vi "GetValueString.vi"(7 "LabVIEW Web Service Request":refnum<class "Web Request.lvclass">, 11 "ControlName":string="Start") -> (1 "Error":i32, 2 "ErrorString":string, 3 "dataOut":string)   [LabVIEW 2024]
uses:
  <vilib>/wsapi/Web Request.lvclass
  g_VIServerPort.vi
panel:
  out "value":string
  out "errorOut":errorcluster
  # "Use the Web Service Request input terminal to call the VIs on the Web Services palette. Do not remove it from the connector pane unless you don't need access to the palette."
  # "Each additional control wired to the connector pane will be available as an input in the URL. To include an indicator in terminal-mode output (the default setting), it must also be wired to the connector pane."
  # "http://127.0.0.1:8002/WebService/GetValueString?ControlName=MPBID_s"
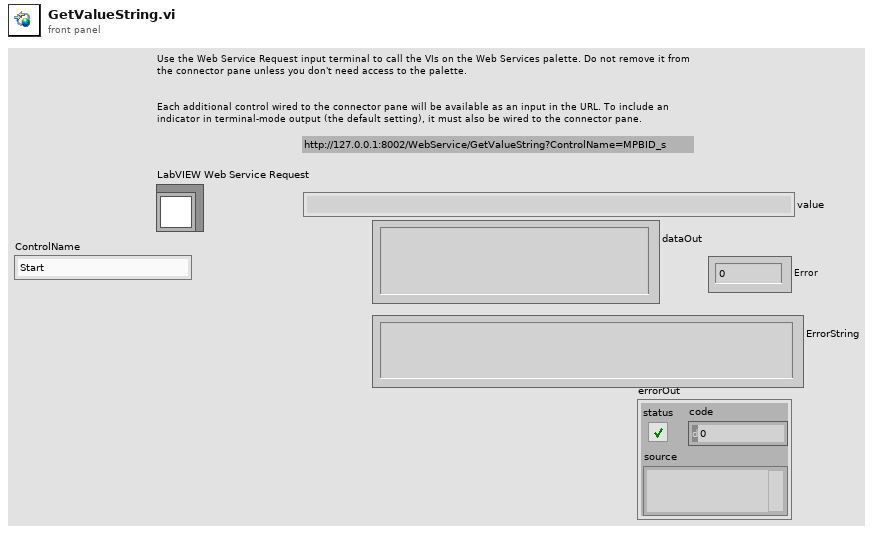
[diagram p1: front panel]
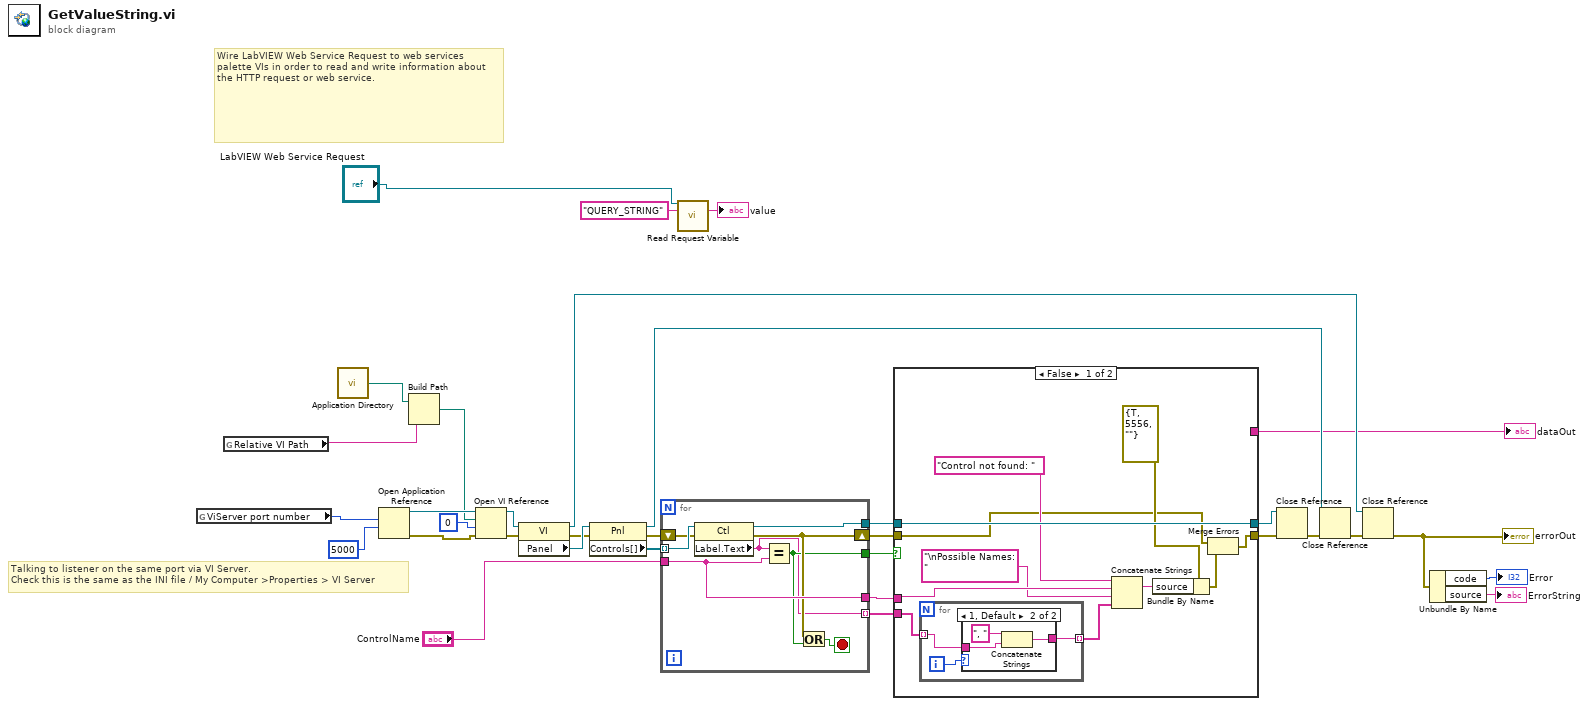
[diagram p0: block diagram]
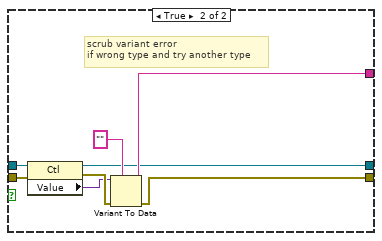
[diagram p3: hidden frame]
diagram:
  # "Talking to listener on the same port via VI Server.\nCheck this is the same as the INI file / My Computer >Properties > VI Server"
  # "Wire LabVIEW Web Service Request to web services palette VIs in order to read and write information about the HTTP request or web service."
  n1 = global read "g_VIServerPort.vi" "ViServer port number"() -> (w2:u16)
  n2 = global read "g_VIServerPort.vi" "Relative VI Path"() -> (w1:string)
  n3 = call <vilib>:"Application Directory.vi"() -> ("Application Directory"=w8:path)
  n4 = Open Application Reference(9:5000 ("timeout ms (60000)"), 10:w2) -> (0:w14:errorcluster, 3:w15:refnum<vi>)  [unwired: 2 in]
  n5 = Build Path(base path=w8, name or relative path=w1) -> (appended path=w7:path)
  n6 = Open VI Reference(application reference (local)=w15, vi path=w7, options=0, error in (no error)=w14) -> (vi reference=w17:refnum<vi>, error out=w29:errorcluster)  [unwired: 2 in]
  n7 = property class="VI"(reference=w17, error in=w29) -> (reference out=w24:refnum<vi>, error out=w28:errorcluster, "Panel"=w32:refnum<vi>)
  n8 = property class="Pnl"(reference=w32, error in=w28) -> (reference out=w18:refnum<vi>, error out=w27:errorcluster, "Controls[]"=w31:refnum<vi>[])
  n9 = for {
    tunnel: w31 -> [w41] mode=indexing
    tunnel: "ControlName" -> [w38]
    tunnel: [w35] -> w26
    tunnel: [w39] -> w19
    tunnel: [w38] -> w16
    shift-right: [w36] -> w20
    shift-left: w27 -> [w40]
    tunnel: [w34] -> w10 mode=indexing
    stop <- w37 stop-if-true
    n10 = property class="Ctl"(reference=w41, error in=w40) -> (reference out=w39:refnum<vi>, error out=w36:errorcluster, "Label.Text"=w34:string)
    n11 = Equal?(x=w34, y=w38) -> (x = y?=w35:bool)
    n12 = Or(x=w36, y=w35) -> (x .or. y?=w37:bool)
  }
  n13 = call <vilib>:"Read Request Variable.vi"("LabVIEW Web Service Request"="LabVIEW Web Service Request", "variable name"="QUERY_STRING") -> ("value"=→"value":string)  [unwired: 11 in, 2 out]
  n14 = case shown="False" w26 {
    tunnel: w19 -> [w52 w67]
    tunnel: [w52 w60] -> w25
    tunnel: [w46 w62] -> w21
    tunnel: w20 -> [w47 w66]
    tunnel: w16 -> [w45 _]
    tunnel: w10 -> [w43 _]
    tunnel: [_ w61] -> w3
    frame False {
      n15 = for {
        tunnel: w43 -> [w53] mode=indexing
        tunnel: [w55] -> w42 mode=indexing
        i -> [w54]
        n16 = case shown="1, Default" w54 {
          tunnel: [w56 w59] -> w55
          tunnel: w53 -> [w56 w57]
          frame 0 {
          }
          frame 1, Default {
            n17 = Concatenate Strings(", " ("string"), w57) -> (w59:string)
          }
        }
      }
      n18 = Concatenate Strings("Control not found: " ("string"), w45, "\nPossible Names: " ("string"), w42) -> (w50:string)
      n19 = Bundle By Name(cluster=errorcluster {"status"=TRUE, "code"=5556, "source"=""} ("error constant"), "source"=w50) -> (w48:errorcluster)
      n20 = Merge Errors(w47, w48) -> (w46:errorcluster)
    }
    frame True {
      # "scrub variant error\nif wrong type and try another type"
      n21 = property class="Ctl"(reference=w67, error in=w66) -> (reference out=w60:refnum<vi>, error out=w65:errorcluster, "Value"=w64:variant)
      n22 = Variant To Data(error in=w65, type="", Variant=w64) -> (data=w61:string, error out=w62:errorcluster)
    }
  }
  "dataOut" <- w3
  n23 = Close Reference(reference=w25, error in (no error)=w21) -> (error out=w23:errorcluster)
  n24 = Close Reference(reference=w18, error in (no error)=w23) -> (error out=w22:errorcluster)
  n25 = Close Reference(reference=w24, error in (no error)=w22) -> (error out=w13:errorcluster)
  "errorOut" <- w13
  n26 = Unbundle By Name(w13) -> ("code"=→"Error":i32, "source"=→"ErrorString":string)
